vi "TestBuildPISLoop.vi"(8 "error in (no error)":errorcluster) -> (0 "error out":errorcluster)   [LabVIEW 2016]
uses:
  <vilib>/addons/_JKI Toolkits/Caraya/classes/Test/Test.lvclass
  <vilib>/addons/_JKI Toolkits/Caraya/classes/Assert/Assert.lvclass
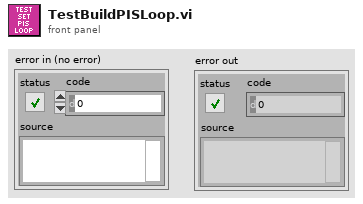
[diagram p1: front panel]
types:
  T1 = cluster{"setpoint":string, "pgain":string, "igain":string, "sgain":string}
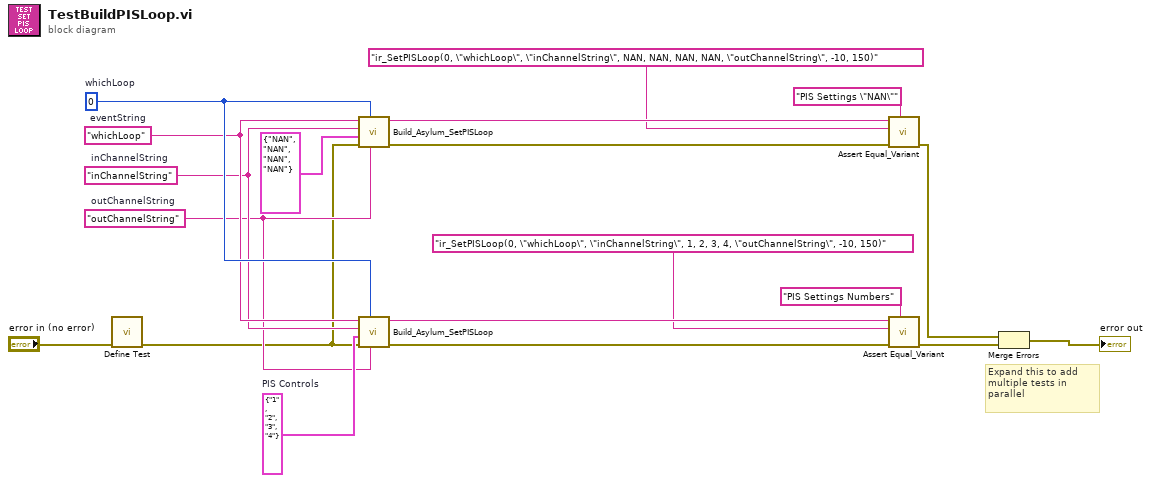
[diagram p0: block diagram]
diagram:
  w2 = "outChannelString"  # outChannelString
  w13 = T1 {"setpoint"="1", "pgain"="2", "igain"="3", "sgain"="4"}  # PIS Controls
  w3 = "inChannelString"  # inChannelString
  w4 = "whichLoop"  # eventString
  w5 = 0  # whichLoop
  # "Expand this to add multiple tests in parallel"
  n1 = call <vilib>:"Define Test.vi"("error in (no error)"="error in (no error)") -> ("error out"=w1:errorcluster)  [unwired: 10 in]
  n2 = call "Build_Asylum_SetPISLoop.vi"("outChannelString"=w2, "whichLoop"=w5, "error in (no error)"=w1, "PIS Controls"=T1 {"setpoint"="NAN", "pgain"="NAN", "igain"="NAN", "sgain"="NAN"}, "inChannelString"=w3, "eventString"=w4) -> ("error out"=w10:errorcluster, "Command"=w11:string)  [unwired: 4 in]
  n3 = call "Build_Asylum_SetPISLoop.vi"("outChannelString"=w2, "whichLoop"=w5, "error in (no error)"=w1, "PIS Controls"=w13, "inChannelString"=w3, "eventString"=w4) -> ("error out"=w15:errorcluster, "Command"=w14:string)  [unwired: 4 in]
  n4 = call <vilib>:"Assert Equal_Variant.vi"("Label"="PIS Settings \"NAN\"", "error in (no error)"=w10, "Y"="ir_SetPISLoop(0, \"whichLoop\", \"inChannelString\", NAN, NAN, NAN, NAN, \"outChannelString\", -10, 150)", "X"=w11) -> ("error out"=w8:errorcluster)  [unwired: 7 in]
  n5 = call <vilib>:"Assert Equal_Variant.vi"("Label"="PIS Settings Numbers", "error in (no error)"=w15, "Y"="ir_SetPISLoop(0, \"whichLoop\", \"inChannelString\", 1, 2, 3, 4, \"outChannelString\", -10, 150)", "X"=w14) -> ("error out"=w17:errorcluster)  [unwired: 7 in]
  n6 = Merge Errors(w8, w17) -> (→"error out":errorcluster)
